vi "LoadWaypoints.vi"(11 "Path Name":string) -> (3 "Waypoints":T1(array[cluster]))   [LabVIEW 2017]
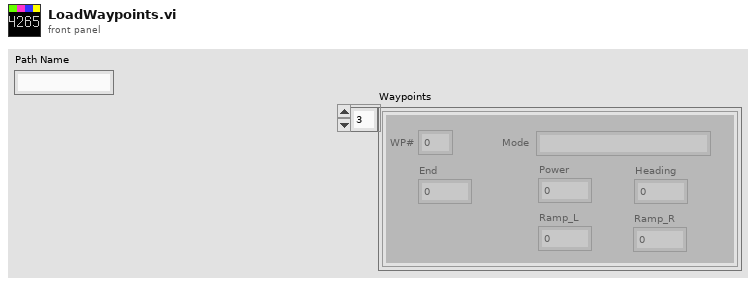
[diagram p1: front panel]
types:
  T1 = cluster{"WP#":i32, "Mode":string, "Power":dbl, "Heading":dbl, "Ramp_L":dbl, "Ramp_R":dbl, "End":dbl}[]
  T2 = cluster{"WP#":i32, "Mode":string, "Power":dbl, "Heading":dbl, "Ramp_L":dbl, "Ramp_R":dbl, "End":dbl}
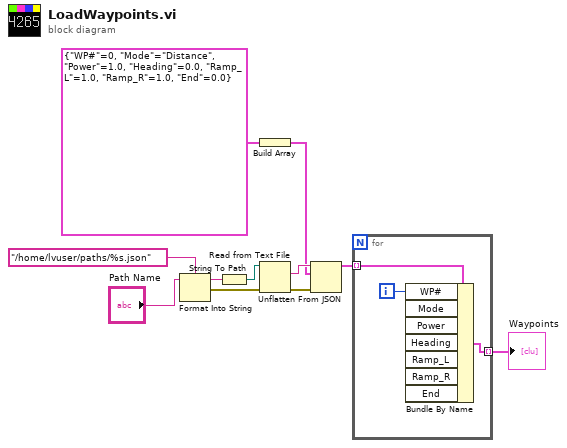
[diagram p0: block diagram]
diagram:
  n1 = Format Into String(format string="/home/lvuser/paths/%s.json", initial string="Path Name") -> (resulting string=w6:string, error out=w5:errorcluster)  [unwired: 2 in]
  n2 = String To Path(string=w6) -> (path=w11:path)
  n3 = Build Array(T2 {"WP#"=0, "Mode"="Distance", "Power"=1.0, "Heading"=0.0, "Ramp_L"=1.0, "Ramp_R"=1.0, "End"=0.0}) -> (w9:T1)
  n4 = Read from Text File(file (use dialog)=w11, error in=w5) -> (text=w10:string, error out=w4:errorcluster)  [unwired: 2 in, 2 out]
  n5 = Unflatten From JSON(JSON string=w10, type and defaults=w9, error in (no error)=w4) -> (value=w3:T1)  [unwired: 4 in, 1 out]
  n6 = for {
    tunnel: w3 -> [w14] mode=indexing
    tunnel: [w13] -> w2 mode=indexing
    i -> [w12]
    n7 = Bundle By Name(cluster=w14, "WP#"=w12) -> (w13:T2)  [unwired: 6 in]
  }
  "Waypoints" <- w2
